vi "attenuator status.vi"(7 "Actions":T1=enum."Clear", 8 "Error In":errorcluster, 10 "i":i32) -> (0 "Error Out":errorcluster, 2 "i":i32)   [LabVIEW 2018]
uses:
  Controls/FGV Actions.ctl
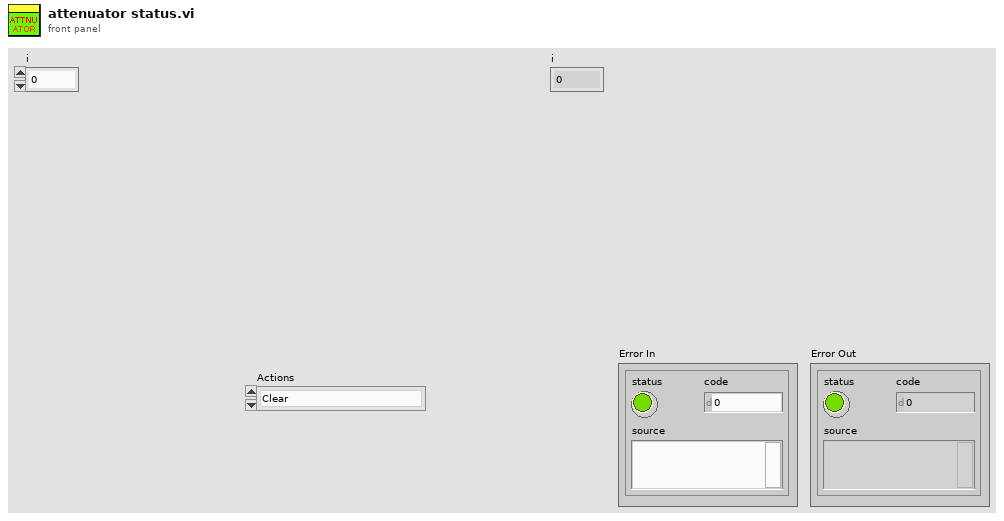
[diagram p1: front panel]
types:
  T1 = typedef "FGV Actions.ctl" = enum16{"Init", "Set", "Get", "Clear"}
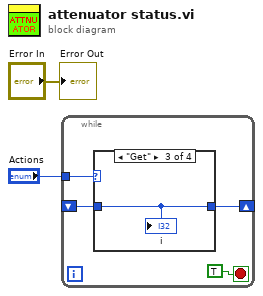
[diagram p0: block diagram]
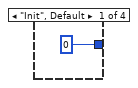
[diagram p2: hidden frame]
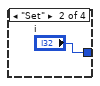
[diagram p3: hidden frame]
diagram:
  n1 = while {
    tunnel: "Actions" -> [w5]
    shift-right: [w4] -> _
    shift-left: _ -> [w3]
    stop <- TRUE stop-if-true
    n2 = case shown="\"Get\"" w5 {
      tunnel: [0 "i" w9 _] -> w4
      tunnel: w3 -> [_ _ w9 _]
      frame "Init", Default {
      }
      frame "Set" {
      }
      frame "Get" {
        "i" <- w9
      }
      frame "Clear" {
      }
    }
  }
  "Error Out" <- "Error In"
